vi "Absolute Angle Difference in Degrees.vi"(9 "angle 2 (deg)":dbl, 11 "angle 1 (deg)":dbl) -> (2 "|angle 1 - angle 2| (deg)":dbl)   [LabVIEW 2017, in "NI_Robotics Utilities.lvlib"]
doc: "This VI is deprecated. Use <vi.lib>\\Analysis\\coordinate.llb\\Absolute Angle Difference.vi instead."
uses:
  <vilib>/robotics/Utilities/NI_Robotics Utilities.lvlib
  <vilib>/robotics/Utilities/Angle Range_Degrees.ctl
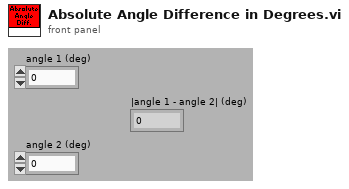
[diagram p1: front panel]
types:
  T1 = typedef "NI_Robotics Utilities.lvlib/Angle Range_Degrees.ctl" = enum16{"none", "-180 to 180", "0 to 360"}
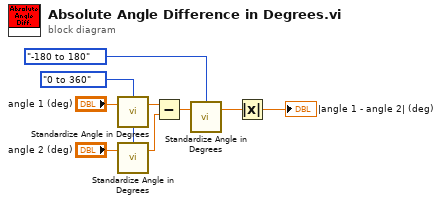
[diagram p0: block diagram]
diagram:
  w2 = Angle_Range_Degrees."0 to 360" ("range (-180 to 180)")
  n1 = call <vilib>:"Standardize Angle in Degrees.vi"("angle in (deg)"="angle 1 (deg)", "range (-180 to 180)"=w2) -> ("angle out (deg)"=w7:dbl)  [unwired: 3 in]
  n2 = call <vilib>:"Standardize Angle in Degrees.vi"("angle in (deg)"="angle 2 (deg)", "range (-180 to 180)"=w2) -> ("angle out (deg)"=w6:dbl)  [unwired: 3 in]
  n3 = Subtract(x=w7, y=w6) -> (x-y=w5:dbl)
  n4 = call <vilib>:"Standardize Angle in Degrees.vi"("angle in (deg)"=w5, "range (-180 to 180)"=Angle_Range_Degrees."-180 to 180") -> ("angle out (deg)"=w4:dbl)  [unwired: 3 in]
  n5 = Absolute Value(x=w4) -> (abs(x)=→"|angle 1 - angle 2| (deg)":dbl)
